vi "Get Abort Requested.vi"(8 "error in (no error)":errorcluster, 11 "refnum in":T1) -> (0 "error out":errorcluster, 2 "AbortRequested":bool, 3 "refnum out":T1)   [LabVIEW 2025, in "xTest.lvlib"]
uses:
  xTest.lvlib
  ContextProxy.ctl
  D:/xTestPlatform/xTestPlatform/bin/x86/Debug/net8.0-windows/win-x86/xTestPlatform.Interop.dll
  xTestPlatform/bin/x86/Debug/net8.0-windows/win-x86/xTestPlatform.Interop.dll
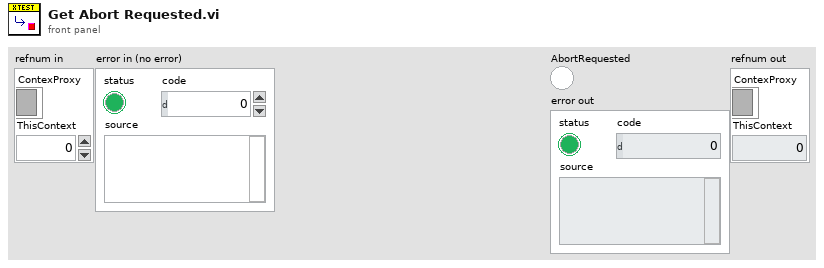
[diagram p1: front panel]
types:
  T1 = typedef "xTest.lvlib/ContextProxy.ctl" = cluster{"ContexProxy":refnum<k39>, "ThisContext":i32}
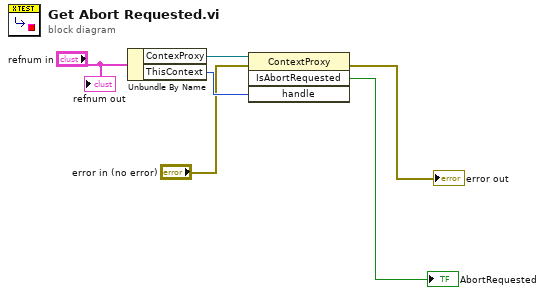
[diagram p0: block diagram]
diagram:
  n1 = Unbundle By Name("refnum in") -> ("ContexProxy"=w5:refnum<k39>, "ThisContext"=w4:i32)
  n2 = invoke class="ContextProxy" method="IsAbortRequested"(reference=w5, error in="error in (no error)", "handle"=w4) -> (error out=→"error out":errorcluster, "IsAbortRequested"=→"AbortRequested":bool)  [unwired: 1 in, 2 out]
  "refnum out" <- "refnum in"
